vi "Send AddShape Event.vi"(7 "Auto-Refresh (T)":bool=TRUE, 8 "error in (no error)":errorcluster, 9 "Backward":bool, 10 "New Shape Reference":refnum<data-value>, 11 "Editor Handler in":refnum<class "Image Editor Handler.lvclass">) -> (0 "error out":errorcluster, 3 "Editor Handler out":refnum<class "Image Editor Handler.lvclass">)   [LabVIEW 2015, in "LV Image Editor Framework.lvlib" / "Image Editor Handler.lvclass"]
uses:
  Image Editor Handler.lvclass
  Forms/Shape/Shape.lvclass
  Image Editor Handler.lvclass/Image Editor Handler.ctl
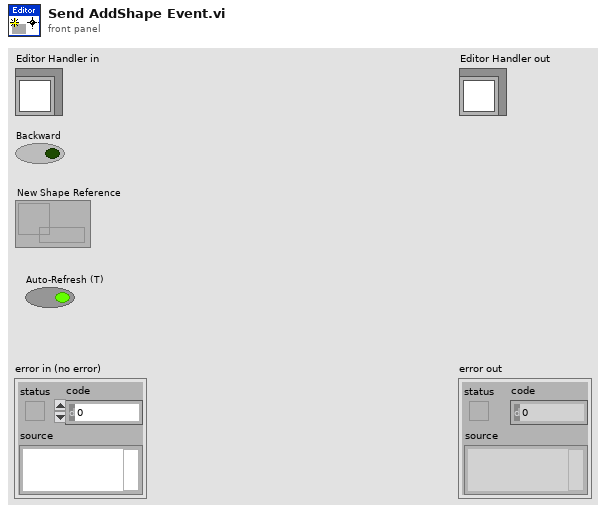
[diagram p1: front panel]
types:
  T1 = cluster{"New Shape Reference":refnum<data-value>, "Backward":bool}
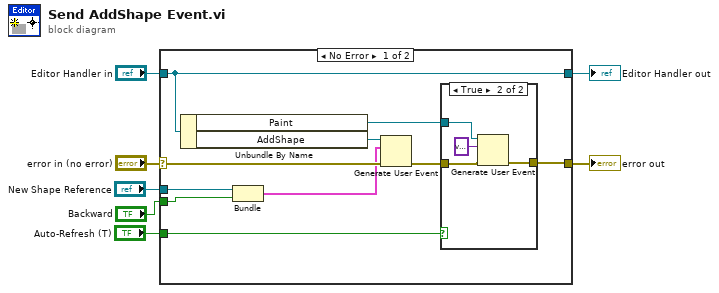
[diagram p0: block diagram]
diagram:
  n1 = case shown="No Error" "error in (no error)" {
    selector: "error in (no error)" -> [w15 w24]
    tunnel: [w8 w24] -> w6
    tunnel: [w17 w23] -> w4
    tunnel: "Editor Handler in" -> [w17 w23]
    tunnel: "New Shape Reference" -> [w14 _]
    tunnel: "Backward" -> [w13 _]
    tunnel: "Auto-Refresh (T)" -> [w11 _]
    frame No Error {
      n2 = Unbundle By Name(w17) -> ("Paint"=w10:refnum<user-event>, "AddShape"=w16:refnum<user-event>)
      n3 = Bundle("New Shape Reference"=w14, "Backward"=w13) -> (w12:T1)  [unwired: 1 in]
      n4 = Generate User Event(user event=w16, event data cluster=w12, error in=w15) -> (error out=w9:errorcluster)  [unwired: 1 in, 1 out]
      n5 = case shown="True" w11 {
        tunnel: w10 -> [_ w22]
        tunnel: w9 -> [w18 w21]
        tunnel: [w18 w20] -> w8
        frame False {
        }
        frame True {
          n6 = Generate User Event(user event=w22, event data cluster=variant ("event data"), error in=w21) -> (error out=w20:errorcluster)  [unwired: 1 in, 1 out]
        }
      }
    }
    frame Error {
    }
  }
  "error out" <- w6
  "Editor Handler out" <- w4
